vi "VI Data to JSON.vi"(7 "Generation options":T1={"Minify?"=FALSE, "Disabled Tabs"=[], "Default Tab"=enum."FP"}, 8 "error in":errorcluster, 11 "VI Path":path) -> (0 "error out":errorcluster, 3 "JSON string":string)   [LabVIEW 2019]
uses:
  <vilib>/Utility/miscctls.llb/LVPositionTypeDef.ctl
  <vilib>/Utility/miscctls.llb/LVBoundsTypeDef.ctl
  Typedefs/FP Data.ctl
  Typedefs/BD Data.ctl
  Typedefs/VI Data.ctl
  Typedefs/VI Metadata.ctl
  Typedefs/Diagram Group.ctl
  Typedefs/Diagram to Structure.ctl
  Typedefs/Structure to Diagram.ctl
  Typedefs/Tab.ctl
  Typedefs/Options.ctl
  Typedefs/Generation options.ctl
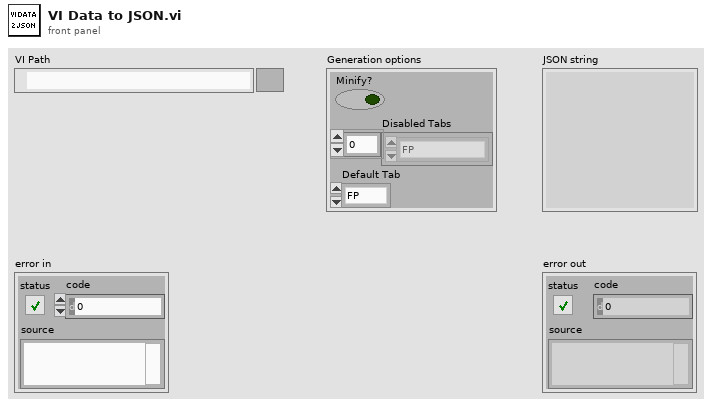
[diagram p1: front panel]
types:
  T1 = typedef "Generation options.ctl" = cluster{"Minify?":bool, "Disabled Tabs":T2[], "Default Tab":T2}
  T2 = typedef "Tab.ctl" = enum16{"Info", "FP", "BD"}
  T3 = typedef "VI Data.ctl" = cluster{"FP":T4, "BD":T7, "Metadata":T11, "Options":T12}
  T4 = typedef "FP Data.ctl" = cluster{"Bounds":T5, "Position":T6, "Color":string, "Image":string, "Page to PageSelectors":cluster{"PageSelector":cluster{"Page Index":i32, "UID":i32}, "PageSelector UID":i32[]}[], "PageSelector to Pages":cluster{"UID":i32, "PageSelector Data":cluster{"Page Images":string[], "Default Page":u32, "Position":T6, "Bounds":T5}}[]}
  T5 = typedef "LVBoundsTypeDef.ctl" = cluster{"Width":u32, "Height":u32}
  T6 = typedef "LVPositionTypeDef.ctl" = cluster{"Left":i32, "Top":i32}
  T7 = typedef "BD Data.ctl" = cluster{"Bounds":T5, "Position":T6, "Color":string, "Image":string, "Structure to Diagram":T8, "Diagram to Structure":T10, "TLD UID":i32}
  T8 = typedef "Structure to Diagram.ctl" = cluster{"UID":i32, "Diagram Group":T9}[]
  T9 = typedef "Diagram Group.ctl" = cluster{"Diagram Data":cluster{"UID":i32, "Diagram Image":string}[], "Position":T6, "Bounds":T5, "Default Frame":u32}
  T10 = typedef "Diagram to Structure.ctl" = cluster{"Diagram UID":i32, "Diagram Children":i32[]}[]
  T11 = typedef "VI Metadata.ctl" = cluster{"Image":string, "Description":string, "VI Name":string, "VI Version":string}
  T12 = typedef "Options.ctl" = cluster{"Disabled Tabs":string[], "Default Tab":string}
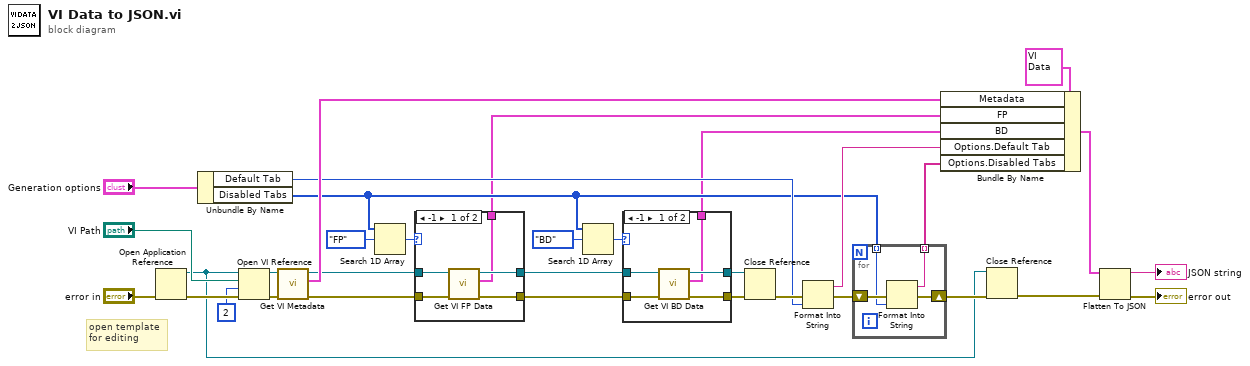
[diagram p0: block diagram]
diagram:
  # "open template\nfor editing"
  n1 = Open Application Reference(8:"error in") -> (0:w30:errorcluster, 3:w2:refnum<vi>)  [unwired: 3 in]
  n2 = Unbundle By Name("Generation options") -> ("Default Tab"=w12:T2, "Disabled Tabs"=w9:T2[])
  n3 = Open VI Reference(application reference (local)=w2, vi path="VI Path", options=2, error in (no error)=w30) -> (vi reference=w4:refnum<vi>, error out=w28:errorcluster)  [unwired: 2 in]
  n4 = call "Get VI Metadata.vi"("error in"=w28, "VI ref in"=w4) -> ("error out"=w24:errorcluster, "Metadata"=w27:T11, "VI ref out"=w23:refnum<vi>)  [unwired: 7 in]
  n5 = Search 1D Array(1D array=w9, element=Tab."FP") -> (index of element=w17:i32)  [unwired: 1 in]
  n6 = case shown="-1" w17 {
    tunnel: w24 -> [w38 w39]
    tunnel: w23 -> [w37 w40]
    tunnel: [w36 w39] -> w21
    tunnel: [w35 w40] -> w20
    tunnel: [w34 _] -> w6
    frame -1 {
      n7 = call "Get VI FP Data.vi"("error in"=w38, "VI ref in"=w37) -> ("error out"=w36:errorcluster, "FP Data"=w34:T4, "VI ref out"=w35:refnum<vi>)  [unwired: 7 in]
    }
    frame Default {
    }
  }
  n8 = Search 1D Array(1D array=w9, element=Tab."BD") -> (index of element=w16:i32)  [unwired: 1 in]
  n9 = case shown="-1" w16 {
    tunnel: [w45 w47] -> w22
    tunnel: w21 -> [w44 w47]
    tunnel: w20 -> [w43 w46]
    tunnel: [w42 w46] -> w19
    tunnel: [w41 _] -> w7
    frame -1 {
      n10 = call "Get VI BD Data.vi"("error in"=w44, "VI ref in"=w43) -> ("error out"=w45:errorcluster, "BD"=w41:T7, "VI ref out"=w42:refnum<vi>)  [unwired: 7 in]
    }
    frame Default {
    }
  }
  n11 = Close Reference(reference=w19, error in (no error)=w22) -> (error out=w13:errorcluster)
  n12 = Format Into String(error in=w13, w12) -> (resulting string=w11:string, error out=w10:errorcluster)  [unwired: 2 in]
  n13 = for {
    tunnel: w9 -> [w50] mode=indexing
    shift-right: [w49] -> w5
    shift-left: w10 -> [w51]
    tunnel: [w48] -> w8 mode=indexing
    n14 = Format Into String(error in=w51, w50) -> (resulting string=w48:string, error out=w49:errorcluster)  [unwired: 2 in]
  }
  n15 = Bundle By Name(cluster=T3 {"FP"={"Bounds"={"Width"=0, "Height"=0}, "Position"={"Left"=0, "Top"=0}, "Color"="", "Image"="", "Page to PageSelectors"=[], "PageSelector to Pages"=[]}, "BD"={"Bounds"={"Width"=0, "Height"=0}, "Position"={"Left"=0, "Top"=0}, "Color"="", "Image"="", "Structure to Diagram"=[], "Diagram to Structure"=[], "TLD UID"=0}, "Metadata"={"Image"="", "Description"="", "VI Name"="", "VI Version"=""}, "Options"={"Disabled Tabs"=[], "Default Tab"=""}} ("Output cluster"), "Metadata"=w27, "FP"=w6, "BD"=w7, "Options.Default Tab"=w11, "Options.Disabled Tabs"=w8) -> (w32:T3)
  n16 = Close Reference(reference=w2, error in (no error)=w5) -> (error out=w3:errorcluster)
  n17 = Flatten To JSON(anything=w32, error in (no error)=w3) -> (JSON string=→"JSON string":string, 11:→"error out":errorcluster)  [unwired: 1 in]
